vi "DTACQ - Write List of Detailed Commands to Text File.vi"(8 "error in":errorcluster, 9 "File Path":path, 10 "Port":u16, 11 "Address":string) -> (0 "error out":errorcluster)   [LabVIEW 2017, in "Communications Library.lvlib"]
doc: "Saves a detailed list of avilable commands to a tab seperated values file.\nThe \"help2\" command is used to retrieve the list of commands.\n\nNote: \nThe help2 command does not list every available command; only commands with detailed help are listed\nA header is prepended to the tab seperated file, giving a desription of each column."
uses:
  Communications Library.lvlib
  <vilib>/Utility/file.llb/Write Delimited Spreadsheet (string).vi
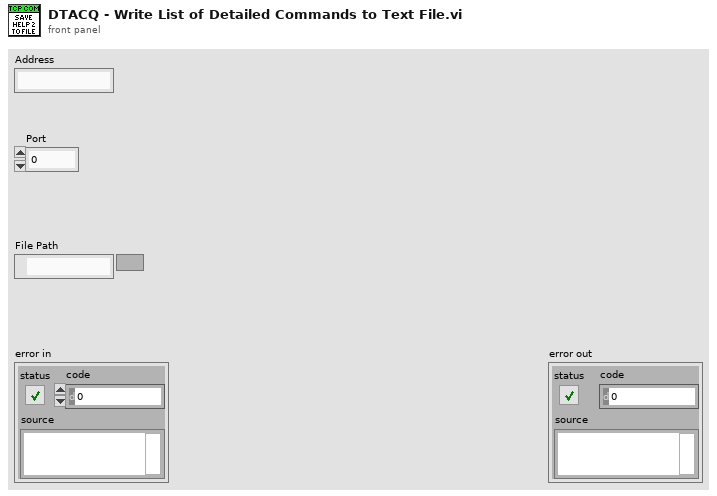
[diagram p1: front panel]
types:
  T1 = typedef "Communications Library.lvlib/DTACQ Connection Data--Cluster.ctl" = cluster{"Description":string, "Address":string, "Port":u16, "timeout (ms)":i32, "Termination Character":string, "TCP Connection Reference":refnum<k5>, "Open Connection":bool}
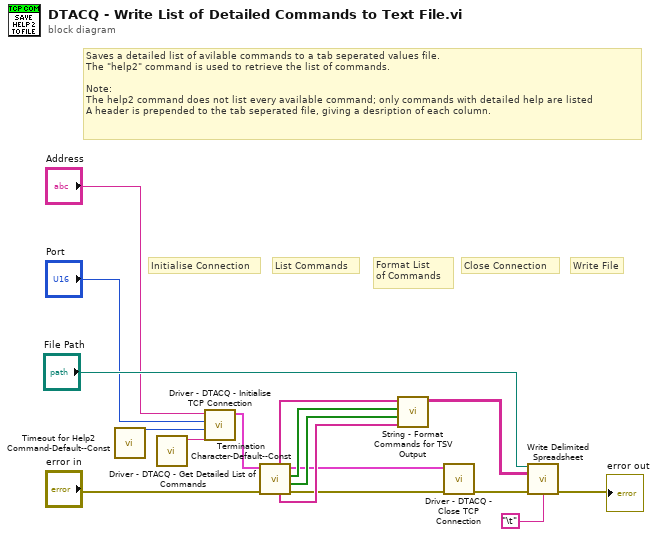
[diagram p0: block diagram]
diagram:
  # "Format List\nof Commands"
  # "Write File"
  # "Close Connection"
  # "List Commands"
  # "Initialise Connection"
  # "Saves a detailed list of avilable commands to a tab seperated values file.\nThe \"help2\" command is used to retrieve the list of commands.\n\nNote: \nThe help2 command does not list every available command; only commands with detailed help are listed\nA header is prepended to the tab seperated file, giving a desription of each column."
  n1 = call "Timeout for Help2 Command-Default--Const.vi"() -> ("timeout (ms)"=w6:i32)  [unwired: 11 in]
  n2 = call "Termination Character-Default--Const.vi"() -> ("Termination Character"=w5:string)  [unwired: 11 in]
  n3 = call "Driver - DTACQ - Initialise TCP Connection.vi"("Termination Character"=w5, "timeout (ms)"=w6, "Port"="Port", "Address"="Address") -> ("DTACQ Connection Data Out"=w4:T1)  [unwired: 7 in]
  n4 = call "Driver - DTACQ - Get Detailed List of Commands.vi"("error in"="error in", "DTACQ Connection Data In"=w4) -> ("error out"=w9:errorcluster, "Write Access"=w15:bool[], "Read Access"=w16:bool[], "DTACQ Connection Data Out"=w10:T1, "Command Descriptions"=w14:string[], "Commands"=w17:string[])  [unwired: 4 in]
  n5 = call "String - Format Commands for TSV Output.vi"("Description"=w14, "Write Access"=w15, "Read Access"=w16, "Command"=w17) -> ("Formatted Array"=w13:string[][])  [unwired: 7 in]
  n6 = call "Driver - DTACQ - Close TCP Connection.vi"("error in"=w9, "DTACQ Connection Data In"=w10) -> ("error out"=w2:errorcluster)  [unwired: 8 in, 1 out]
  n7 = call-poly <vilib>:"Write Delimited Spreadsheet.vi"("file path (dialog if empty)"="File Path", "2D data"=w13, "error in (no error)"=w2, "delimiter (\\t)"="\t") -> ("error out"=→"error out":errorcluster)  [unwired: 10 in, 1 out]
